vi "PCO_Quit.vi"(8 "error in":errorcluster, 10 "Array":i16[](array[numeric]), 11 "ph":u64) -> (3 "Indicator":bool)   [LabVIEW 2014]
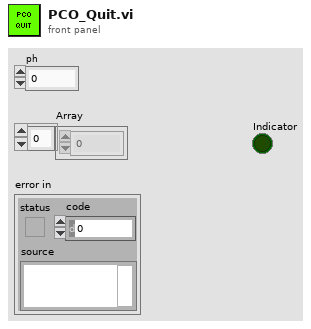
[diagram p1: front panel]
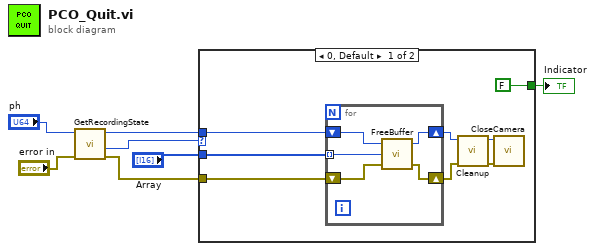
[diagram p0: block diagram]
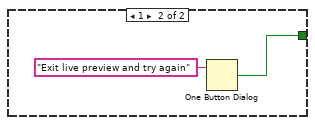
[diagram p2: hidden frame]
diagram:
  n1 = call "GetRecordingState.vi"("ErrorIn"="error in", "ph"="ph") -> ("ErrorOut"=w3:errorcluster, "RecordingState"=w6:u16, "hout"=w5:u64)  [unwired: 2 in, 1 out]
  n2 = case shown="0, Default" w6 {
    tunnel: w5 -> [w15 _]
    tunnel: w3 -> [w14 _]
    tunnel: "Array" -> [w13 _]
    tunnel: [FALSE ("true") w21] -> w1
    frame 0, Default {
      n3 = for {
        shift-right: [w19] -> w11
        shift-left: w15 -> [w20]
        shift-right: [w17] -> w10
        shift-left: w14 -> [w18]
        tunnel: w13 -> [w16] mode=indexing
        n4 = call "FreeBuffer.vi"("error in (no error)"=w18, "BuffNr"=w16, "ph"=w20) -> ("error out"=w17:errorcluster, "hout"=w19:u64)  [unwired: 1 out]
      }
      n5 = call "Cleanup.vi"("error in (no error)"=w10, "ph"=w11) -> ("error out"=w8:errorcluster, "hout"=w9:u64)  [unwired: 8 in]
      n6 = call "CloseCamera.vi"("ErrorIn"=w8, "Handle in"=w9) -> ()  [unwired: 1 in, 3 out]
    }
    frame 1 {
      n7 = One Button Dialog(message="Exit live preview and try again") -> (true=w21:bool)  [unwired: 1 in]
    }
  }
  "Indicator" <- w1
